vi "ReadFileLocations.vi"(8 "error in (no error)":errorcluster, 11 "Model in":refnum<class "Model.lvclass">) -> (0 "error out":errorcluster, 2 "ActuatorLocationPath":T1, 3 "Model out":refnum<class "Model.lvclass">)   [LabVIEW 2016, in "Model.lvclass"]
uses:
  Model.lvclass
  Typedefs/ActuatorLocationPath.ctl
  Model.lvclass/Model.ctl
  Settings/Settings.lvclass
  Typedefs/M1M3SupportEUI_TypeDefs.lvlib
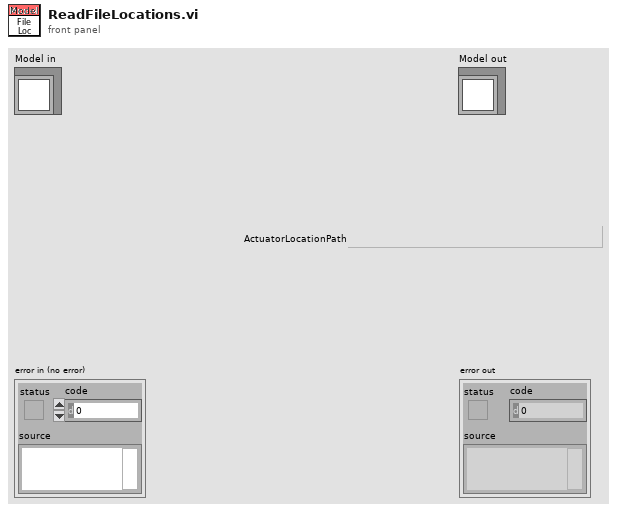
[diagram p1: front panel]
types:
  T1 = typedef "M1M3SupportEUI_TypeDefs.lvlib/ActuatorLocationPath.ctl" = path
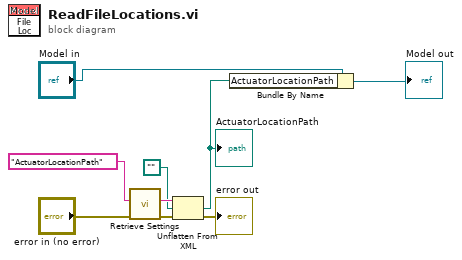
[diagram p0: block diagram]
diagram:
  n1 = call "Retrieve Settings.vi"("error in (no error)"="error in (no error)", "configName"="ActuatorLocationPath") -> ("error out"=w5:errorcluster, "xmlConfig"=w8:string)  [unwired: 7 in, 1 out]
  n2 = Unflatten From XML(xml string=w8, type=T1 path "" ("ActuatorLocationPath"), error in (no error)=w5) -> (value=w2:T1, error out=→"error out":errorcluster)
  "ActuatorLocationPath" <- w2
  n3 = Bundle By Name(cluster="Model in", "ActuatorLocationPath"=w2) -> (→"Model out":refnum<class "Model.lvclass">)
